vi "ImageSubset2RPhiArray (SubVI).vi"(8 "error in (no error)":errorcluster, 9 "Multiplier for Radius":dbl=1.25 format="%#_13g", 10 "Fitted Circle":T2, 11 "Full Image in":T1) -> (0 "error out":errorcluster, 1 "2D Array: r, phi, intensity":dbl[][](array[numeric]), 2 "Radius (Pixels)":dbl, 3 "Subset image out":T1)   [LabVIEW 2016]
uses:
  <vilib>/vision/Image Controls.llb/IMAQ Image.ctl
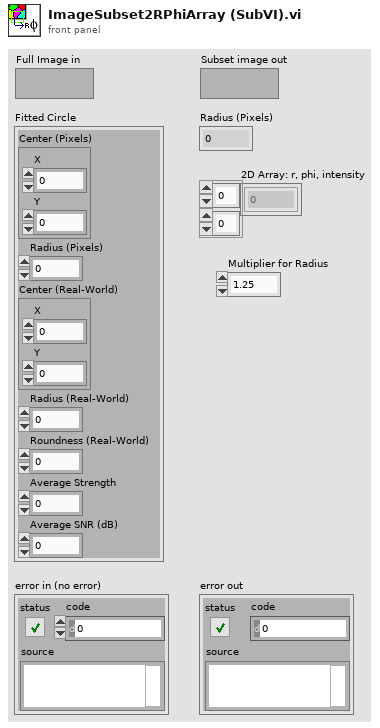
[diagram p1: front panel]
types:
  T1 = typedef "IMAQ Image.ctl" = refnum<image>
  T2 = cluster{"Center (Pixels)":cluster{"X":sgl, "Y":sgl}, "Radius (Pixels)":dbl, "Center (Real-World)":cluster{"X":sgl, "Y":sgl}, "Radius (Real-World)":dbl, "Roundness (Real-World)":dbl, "Average Strength":dbl, "Average SNR (dB)":dbl}
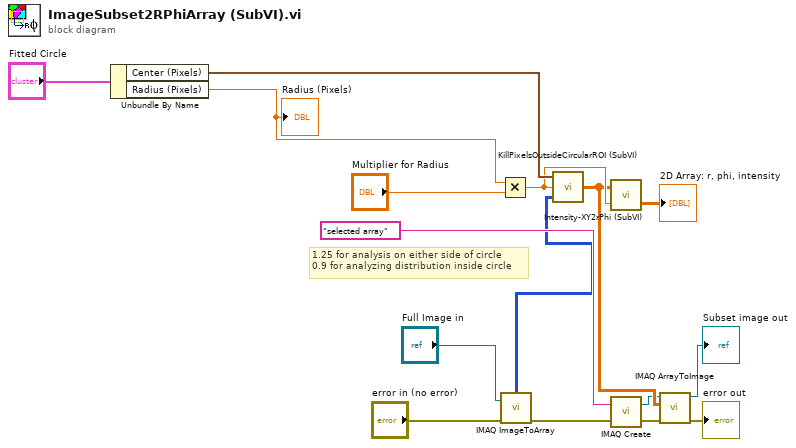
[diagram p0: block diagram]
diagram:
  # "1.25 for analysis on either side of circle\n0.9 for analyzing distribution inside circle"
  n1 = Unbundle By Name("Fitted Circle") -> ("Center (Pixels)"=w15:cluster{"X":sgl, "Y":sgl}, "Radius (Pixels)"=w14:dbl)
  "Radius (Pixels)" <- w14
  n2 = Multiply(x=w14, y="Multiplier for Radius") -> (x*y=w9:dbl)
  n3 = call "IMAQ ImageToArray"("error in (no error)"="error in (no error)", "Image"="Full Image in") -> ("error out"=w11:errorcluster, "Image Pixels (U8)"=w4:u8[][])  [unwired: 2 in, 3 out]
  n4 = call "KillPixelsOutsideCircularROI (SubVI).vi"("XY Array"=w4, "Radius*ScaleFactor"=w9, "Center (Pixels)"=w15) -> ("subarray"=w7:dbl[][])
  n5 = call "Intensity-XY2rPhi (SubVI).vi"("Radius*Scale Factor"=w9, "XY Array"=w7) -> ("2D Array: r, phi, intensity"=→"2D Array: r, phi, intensity":dbl[][])  [unwired: 1 out]
  n6 = call "IMAQ Create"("Image Name"="selected array", "error in (no error)"=w11) -> ("New Image"=w6:T1, "error out"=w12:errorcluster)  [unwired: 3 in]
  n7 = call "IMAQ ArrayToImage"("error in (no error)"=w12, "Image Pixels (U8)"=w7, "Image"=w6) -> ("error out"=→"error out":errorcluster, "Image Out"=→"Subset image out":T1)  [unwired: 7 in]
